vi "Initialize Transfer Groups.vi"(7 "component name":string, 8 "error in (no error)":errorcluster, 10 "Group Configurations":refnum<class "Group Configuration.lvclass">[](array[class]), 11 "UDP Transceiver in":refnum<class "UDP Transceiver.lvclass">) -> (0 "error out":errorcluster, 3 "UDP Transceiver out":refnum<class "UDP Transceiver.lvclass">)   [LabVIEW 2017, in "UDP.lvlib" / "UDP Transceiver.lvclass"]
uses:
  UDP Transceiver.lvclass
  DSF Core.lvlibp/Classes/Configuration/Core/Group/Group Configuration.lvclass
  Transfer Group Parameters.ctl
  Transfer Parameters.ctl
  UDP Transceiver.lvclass/UDP Transceiver.ctl
  DSF Core.lvlibp/Classes/Configuration/Core/Core Configuration.lvclass
  C:/Git/DSF/Components/DSF Core.lvlibp/Classes/Configuration/Core/Core Configuration.lvclass
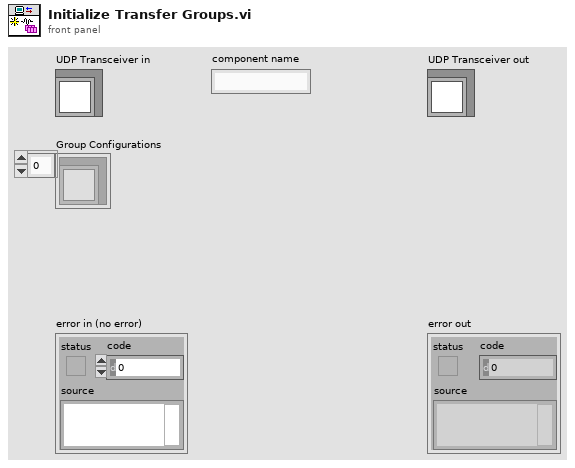
[diagram p1: front panel]
types:
  T1 = typedef "UDP.lvlib/UDP Transceiver.lvclass/Transfer Group Parameters.ctl" = cluster{"transfers":T2[], "max size":i32, "timeout":i32}
  T2 = typedef "UDP.lvlib/UDP Transceiver.lvclass/Transfer Parameters.ctl" = cluster{"group offset":u64, "size":u64, "address":u32, "port":u16}
  T3 = typedef "DSF Core.lvlibp/Group Configuration.lvclass/Core Group Configuration.ctl" = cluster{"name":string, "direction":T4, "cycle timing":T5, "timeout behavior":T6, "enable conversion":bool}
  T4 = typedef "DSF Core.lvlibp/DSF Direction.ctl" = enum8{"Tx", "Rx"}
  T5 = typedef "DSF Core.lvlibp/DSF Timing Info.ctl" = cluster{"priority":u64, "decimation":u64, "offset":u64}
  T6 = typedef "DSF Core.lvlibp/DSF Timeout Behavior.ctl" = enum8{"Increment Late Count", "Throw Error"}
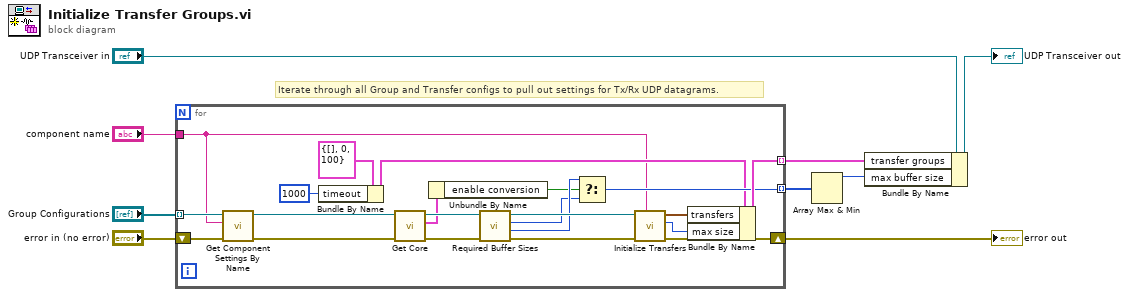
[diagram p0: block diagram]
diagram:
  # "Iterate through all Group and Transfer configs to pull out settings for Tx/Rx UDP datagrams."
  n1 = for {
    tunnel: "Group Configurations" -> [w21] mode=indexing
    shift-right: [w30] -> w8
    shift-left: "error in (no error)" -> [w23]
    tunnel: [w20] -> w6 mode=indexing
    tunnel: [w28] -> w5 mode=indexing
    tunnel: "component name" -> [w10]
    n2 = call "Get Component Settings By Name.vi"("error in (no error)"=w23, "component name"=w10, "Runtime Configuration in"=w21) -> ("error out"=w16:errorcluster, "Runtime Configuration out"=w15:refnum<class "Group Configuration.lvclass">)  [unwired: 6 in, 1 out]
    n3 = Bundle By Name(cluster=T1 {"transfers"=[], "max size"=0, "timeout"=100} ("Rx/Tx Parameters"), "timeout"=1000) -> (w17:T1)
    n4 = call "Get Core.vi"("error in (no error)"=w16, "Group Configuration in"=w15) -> ("error out"=w13:errorcluster, "core"=w12:T3, "Group Configuration out"=w14:refnum<class "Group Configuration.lvclass">)  [unwired: 7 in]
    n5 = Unbundle By Name(w12) -> ("enable conversion"=w11:bool)
    n6 = call-dynamic "Required Buffer Sizes.vi"("error in (no error)"=w13, "Group Configuration in"=w14) -> ("error out"=w27:errorcluster, "string size"=w19:u64, "engine size"=w18:u64, "Group Configuration out"=w26:refnum<class "Group Configuration.lvclass">)  [unwired: 6 in]
    n7 = Select(t=w19, s=w11, f=w18) -> (s? t:f=w20:u64)
    n8 = call "Initialize Transfers.vi"("component name"=w10, "error in (no error)"=w27, "Group Configuration"=w26) -> ("error out"=w30:errorcluster, "max buffer size"=w25:u64, "transfer parameters"=w29:T2[])  [unwired: 6 in]
    n9 = Bundle By Name(cluster=w17, "transfers"=w29, "max size"=w25) -> (w28:T1)
  }
  "error out" <- w8
  n10 = Array Max & Min(array=w6) -> (max value=w2:u64)  [unwired: 3 out]
  n11 = Bundle By Name(cluster="UDP Transceiver in", "transfer groups"=w5, "max buffer size"=w2) -> (→"UDP Transceiver out":refnum<class "UDP Transceiver.lvclass">)
